vi "vibrate_triangle.vi"() -> ()   [LabVIEW 2014]
panel:
  in  "Initial duty cycle":dbl
  in  "Max duty cycle":dbl
  in  "Min duty cycle":dbl
  in  "period (frames)":dbl
  in  "Frequency (Hz)":dbl
  in  "Frames":i32
  in  "Transfer and Run Date Folder After Experiment":bool
  in  "SSH user name":string
  in  "SSH password":string
  in  "Wait before recording (s)":dbl
  in  "Tags":string
  in  "Start Recording":bool
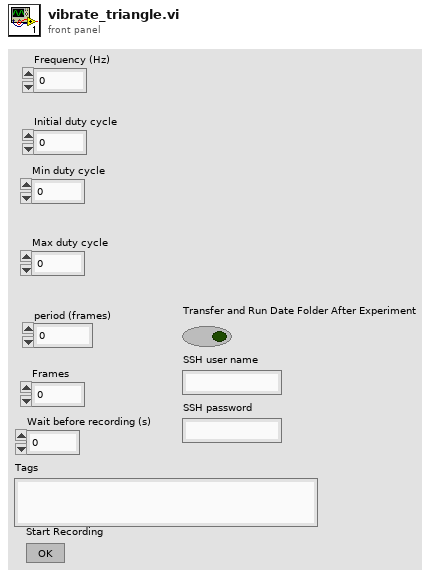
[diagram p1: front panel]
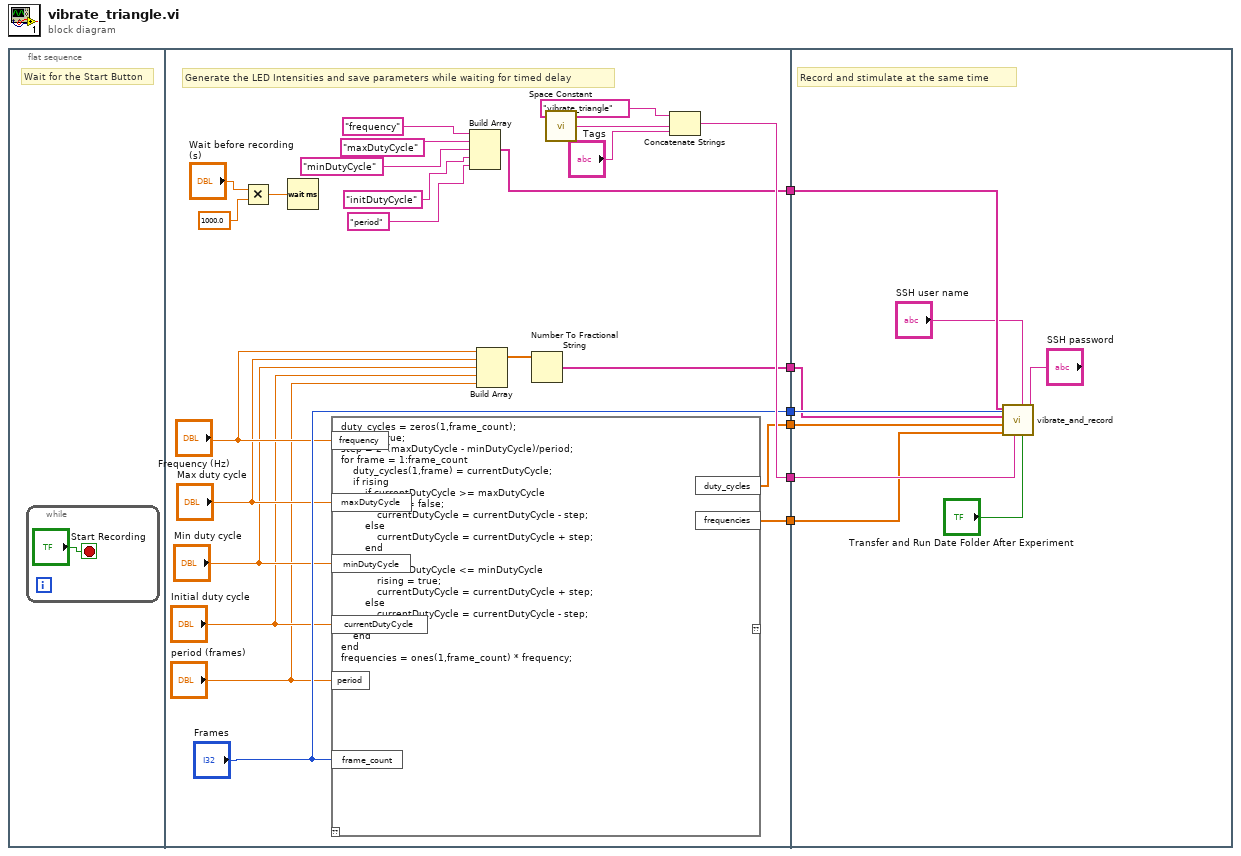
[diagram p0: block diagram]
diagram:
  n1 = flat-sequence {
    tunnel: [w27] -> w6
    tunnel: [w20] -> w5
    tunnel: ["Frames"] -> w4
    tunnel: [w16] -> w3
    tunnel: [w9] -> w2
    tunnel: [w8] -> w1
    tunnel: w6 -> [w39]
    tunnel: w5 -> [w38]
    tunnel: w4 -> [w34]
    tunnel: w3 -> [w33]
    tunnel: w2 -> [w32]
    tunnel: w1 -> [w31]
    frame #0 {
      # "Wait for the Start Button"
      n2 = while {
        stop <- "Start Recording" stop-if-true
      }
    }
    frame #1 {
      # "Generate the LED Intensities and save parameters while waiting for timed delay"
      n3 = Multiply(x="Wait before recording (s)", y=1000.0) -> (x*y=w25:dbl)
      n4 = Wait (ms)(milliseconds to wait=w25) -> ()  [unwired: 1 out]
      n5 = script code="duty_cycles = zeros(1,frame_count);\nrising = true;\nstep = 2*(maxDutyCycle - minDutyCycle)/period;\nfor frame = 1:frame_count\n    duty_cycles(1,frame) = currentDutyCycle;\n    if rising\n        if currentDutyCycle >= maxDutyCycle\n            rising = false;\n            currentDutyCycle = currentDutyCycle - step;\n        else\n            currentDutyCycle = currentDutyCycle + step;\n        end\n    else\n        if currentDutyCycle <= minDutyCycle\n            rising = true;\n            currentDutyCycle = currentDutyCycle + step;\n        else\n            currentDutyCycle = currentDutyCycle - step;\n        end\n    end\nend\nfrequencies = ones(1,frame_count) * frequency;"("currentDutyCycle"="Initial duty cycle", "frame_count"="Frames", "minDutyCycle"="Min duty cycle", "maxDutyCycle"="Max duty cycle", "period"="period (frames)", "frequency"="Frequency (Hz)") -> ("duty_cycles"=w9:dbl[], "frequencies"=w8:dbl[])  [unwired: 1 in, 1 out]
      n6 = Build Array("frequency", "maxDutyCycle", "minDutyCycle", "initDutyCycle", "period") -> (w20:string[])
      n7 = Build Array("Frequency (Hz)", "Max duty cycle", "Min duty cycle", "Initial duty cycle", "period (frames)") -> (w15:dbl[])
      n8 = Number To Fractional String(number=w15) -> (F-format string=w16:string[])  [unwired: 3 in]
      n9 = call <vilib>:"Space Constant.vi"() -> ("String"=w29:string)
      n10 = Concatenate Strings("vibrate_triangle", w29, "Tags") -> (w27:string)
    }
    frame #2 {
      # "Record and stimulate at the same time"
      n11 = call "vibrate_and_record.vi"("SSH password"="SSH password", "Transfer and Run Date Folder After Experiment"="Transfer and Run Date Folder After Experiment", "SSH user name"="SSH user name", "Tags"=w39, "Frames"=w34, "frequencies"=w31, "PWM duty cycles"=w32, "parameters"=w33, "parameters headers"=w38) -> ()  [unwired: 3 in]
    }
  }
